vi "network stream reconnect.vi"(8 "error in (no error)":errorcluster, 10 "Settings":T1, 11 "NetworkConnection in":refnum<class "NetworkConnection.lvclass">) -> (0 "error out":errorcluster, 1 "Connected?":bool, 2 "Public Settings":T1, 3 "NetworkConnection out":refnum<class "NetworkConnection.lvclass">)   [LabVIEW 2020]
uses:
  <vilib>/addons/_JKI.lib/Network_Streams_Connection.llb/NetworkConnection.lvclass
  <vilib>/addons/_JKI.lib/Network_Streams_Connection.llb/PublicSettings.ctl
  <vilib>/addons/_JKI.lib/Network_Streams_Connection.llb/NetworkConnection.lvclass/NetworkConnection.ctl
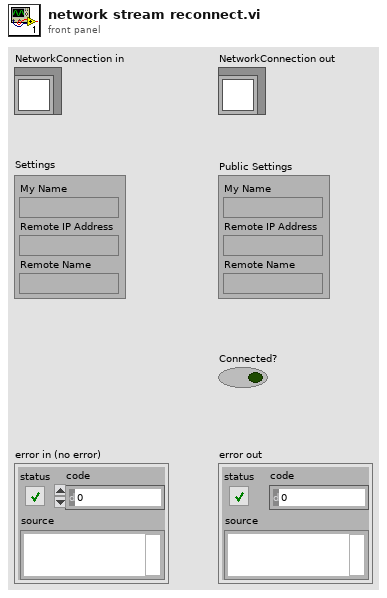
[diagram p1: front panel]
types:
  T1 = typedef "NetworkConnection.lvclass/PublicSettings.ctl" = cluster{"My Name":string, "Remote IP Address":string, "Remote Name":string}
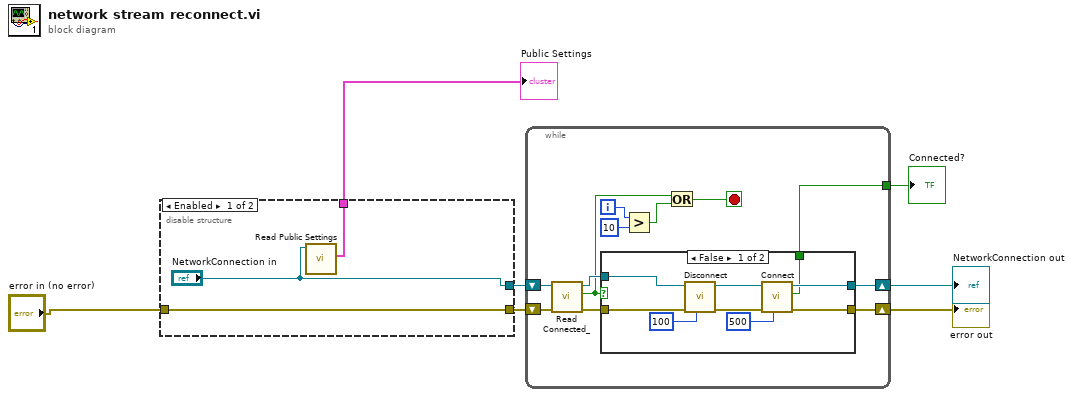
[diagram p0: block diagram]
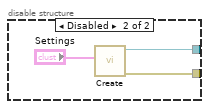
[diagram p2: hidden frame]
diagram:
  n1 = disable-structure shown="Enabled" {
    disable-tunnel: ["NetworkConnection in" w13] -> w3
    disable-tunnel: [w8 w12] -> w4
    disable-tunnel: [w9 _] -> w6
    disable-tunnel: "error in (no error)" -> [w8 _]
    frame Enabled {
      n2 = call <vilib>:"Read Public Settings.vi"("NetworkConnection in"="NetworkConnection in") -> ("Public Settings"=w9:T1)  [unwired: 8 in, 2 out]
    }
    frame Disabled {
      n3 = call <vilib>:"Create.vi"("Settings"="Settings") -> ("error out"=w12:errorcluster, "NetworkConnection out"=w13:refnum<class "NetworkConnection.lvclass">)  [unwired: 9 in]
    }
  }
  "Public Settings" <- w6
  n4 = while {
    shift-right: [w21] -> w2
    shift-left: w3 -> [w25]
    shift-right: [w20] -> w1
    shift-left: w4 -> [w24]
    tunnel: [w14] -> w5
    i -> [w19]
    stop <- w16 stop-if-true
    n5 = call <vilib>:"Read Connected_.vi"("error in (no error)"=w24, "NetworkConnection in"=w25) -> ("error out"=w23:errorcluster, "Connected?"=w15:bool, "NetworkConnection out"=w22:refnum<class "NetworkConnection.lvclass">)  [unwired: 7 in]
    n6 = case shown="False" w15 {
      selector: w15 -> [_ w35]
      tunnel: w23 -> [w30 w36]
      tunnel: w22 -> [w32 w37]
      tunnel: [w33 w37] -> w21
      tunnel: [w34 w36] -> w20
      tunnel: [w26 w35] -> w14
      frame False {
        n7 = call <vilib>:"Disconnect.vi"("Timeout ms (1000)"=100 ("(ms)"), "error in (no error)"=w30, "NetworkConnection in"=w32) -> ("error out"=w29:errorcluster, "NetworkConnection out"=w31:refnum<class "NetworkConnection.lvclass">)  [unwired: 7 in]
        n8 = call <vilib>:"Connect.vi"("Timeout(ms)"=500, "error in (no error)"=w29, "NetworkConnection in"=w31) -> ("error out"=w34:errorcluster, "Connected?"=w26:bool, "NetworkConnection out"=w33:refnum<class "NetworkConnection.lvclass">)  [unwired: 6 in]
      }
      frame True {
      }
    }
    n9 = Greater?(x=w19, y=10) -> (0:w17:bool)
    n10 = Or(x=w15, y=w17) -> (x .or. y?=w16:bool)
  }
  "Connected?" <- w5
  "NetworkConnection out" <- w2
  "error out" <- w1
